vi "MAIN - TLB` Springboard Tool.vi"() -> ()   [LabVIEW 2014, in "TLB` Springboard.lvlib"]
uses:
  TLB` Springboard.lvlib
  Components/State Declaration.ctl
  Components/System Triggers.ctl
  <vilib>/Utility/error.llb/DialogTypeEnum.ctl
  <vilib>/NI/AMC/Read Termination Message.vi
  <vilib>/NI/AMC/Create Single Message.vi
  <vilib>/NI/AMC/Update Message Routing Info.vi
  <vilib>/NI/AMC/Create Multiple Messages.vi
  Components/TypeDef - SHIFTER - TLB` Springboard.ctl
  <vilib>/NI/AMC/Globals.vi
  <vilib>/NI/AMC/Send Message.vi
  Components/Dependencies.llb/TLB`_Dependencies.lvlib
  <vilib>/NI/AMC/AMC.lvlib
panel:
  in  "Add to Project":u16(ring) items=["< Create In New Project... >"]
  in  "Cancel":bool
  in  "Build":bool
  in  "New TLB Name":string
  in  "Destination Folder":path
  out "error out":errorcluster
  # "TLB` Springboard"
  # "Description"
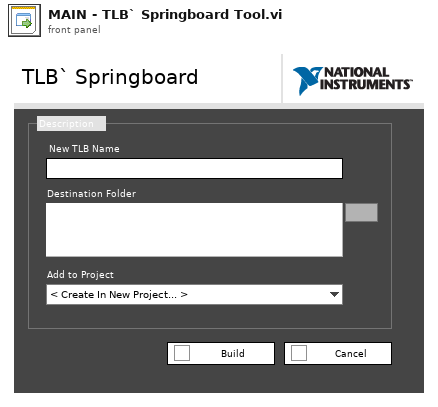
[diagram p1: front panel]
types:
  T1 = typedef "TLB` Springboard.lvlib/System Triggers.ctl" = enum16{"<None>", "Create New", "Cache User Parameters", "Close Application"}
  T2 = typedef "TLB` Springboard.lvlib/State Declaration.ctl" = enum16{"<Startup>", "Idle", "Creating", "<Shutdown>"}
  T3 = enum16{"Clear SR", "Set Display", "Set Shifter", "Initialize Events", "Init Q"}
  T4 = typedef "TLB` Springboard.lvlib/TypeDef - SHIFTER - TLB` Springboard.ctl" = cluster{"State":T2, "User Data":cluster{"New TLB Name":string, "Destination Folder":path, "Project Selection":u16}, "Display Data":cluster{"Active Item Tag":string}, "User Parameter Controls":refnum<vi>[], "Framework Data":cluster{"Exit Event":T5, "Terminate Error":errorcluster}, "Private Data":cluster{"Projects In Memory":refnum<vi>[], "Build Complete":bool}}
  T5 = typedef "TLB` Springboard.lvlib/TLB`_Dependencies.lvlib/Exit Event Ref.ctl" = refnum<user-event>
  T6 = typedef "AMC.lvlib/Message Queue.ctl" = refnum<queue>
  T7 = typedef "DialogTypeEnum.ctl" = enum16{"no dialog", "OK message", "continue or stop message", "auto error handling dialog", "OK message + warnings", "continue/stop + warnings"}
  T8 = enum8{"Enabled", "Disabled", "Disabled and Grayed Out"}
  T9 = enum32{"Invalid", "Standard", "Closed", "Hidden", "Minimized", "Maximized"}
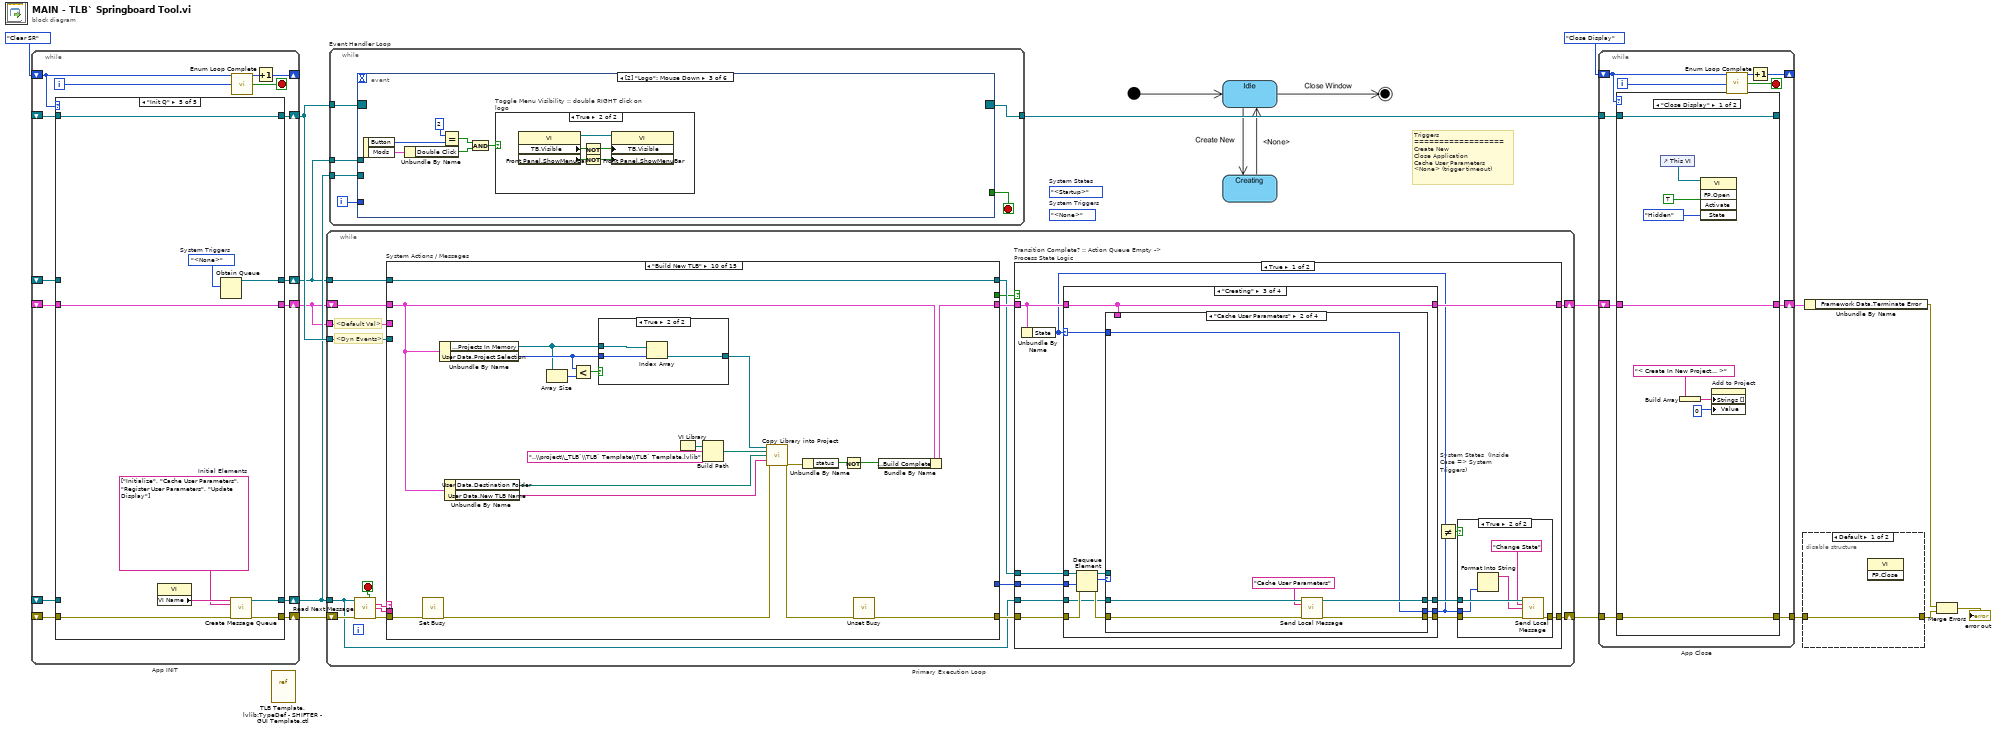
[diagram p0: block diagram]
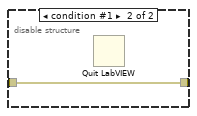
[diagram p2: hidden frame]
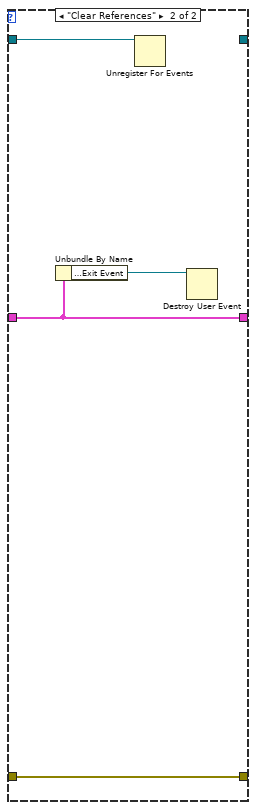
[diagram p3: hidden frame]
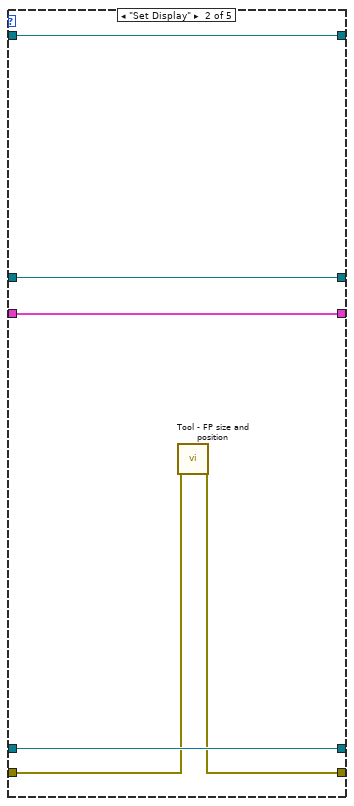
[diagram p5: hidden frame]
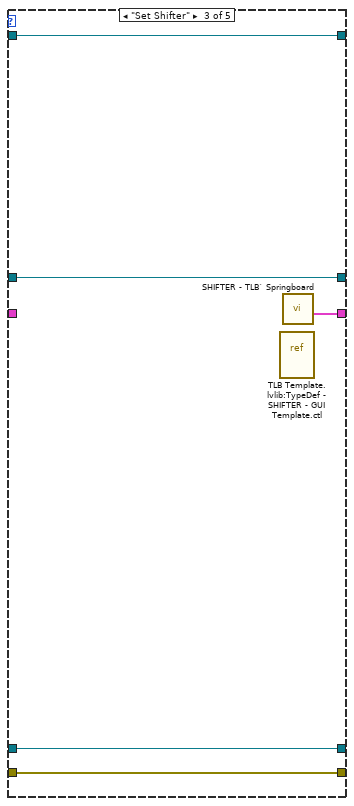
[diagram p6: hidden frame]
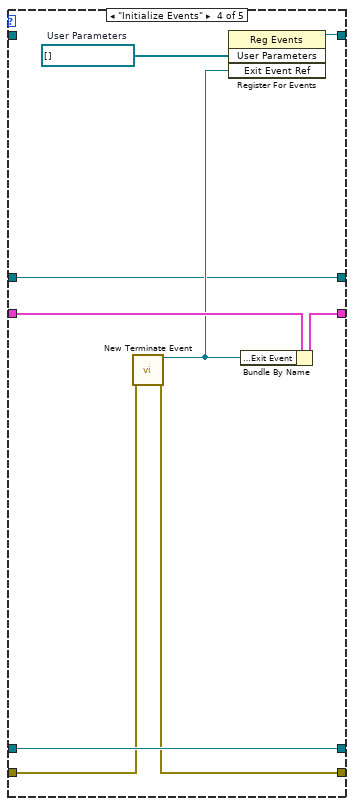
[diagram p7: hidden frame]
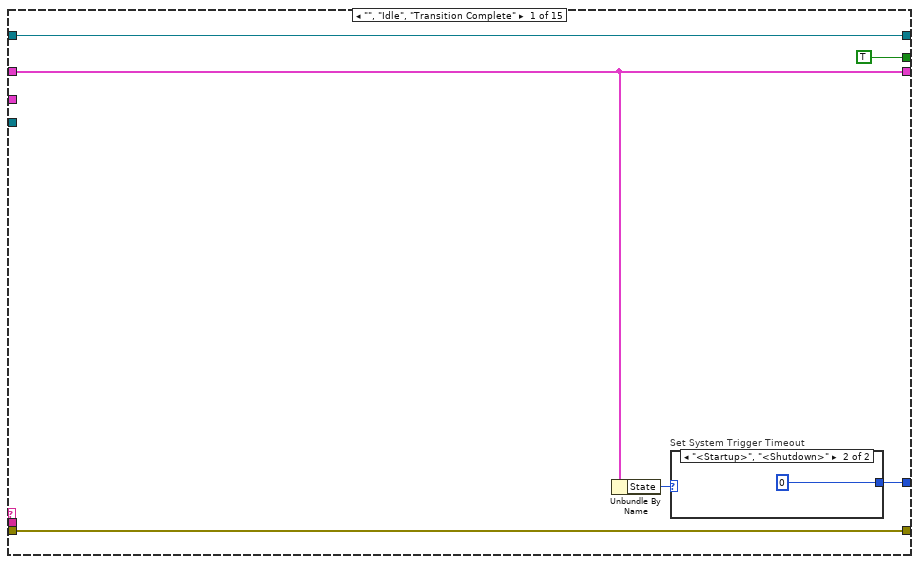
[diagram p8: hidden frame]
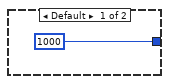
[diagram p9: hidden frame]
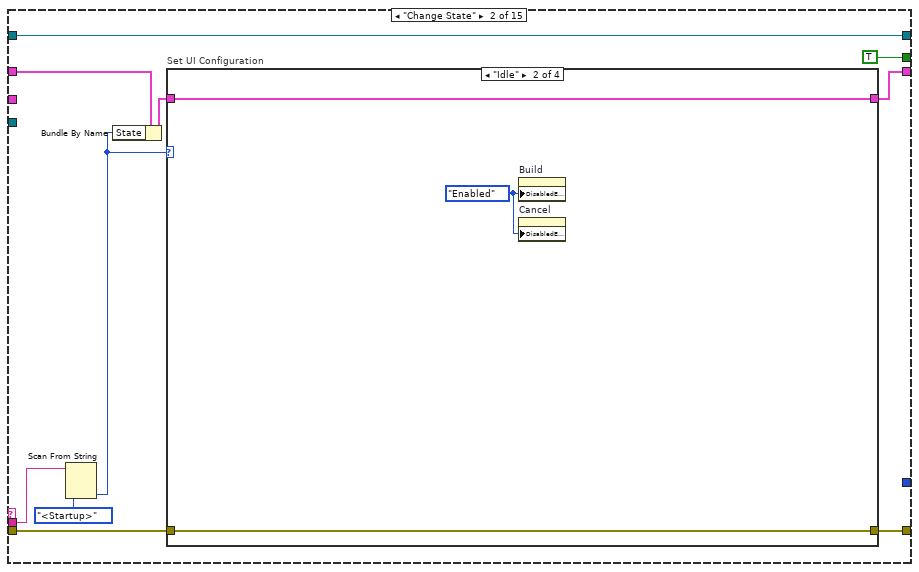
[diagram p10: hidden frame]
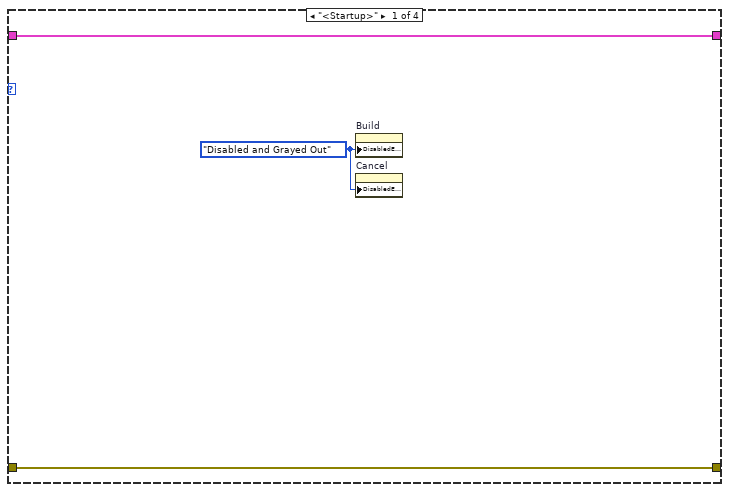
[diagram p11: hidden frame]
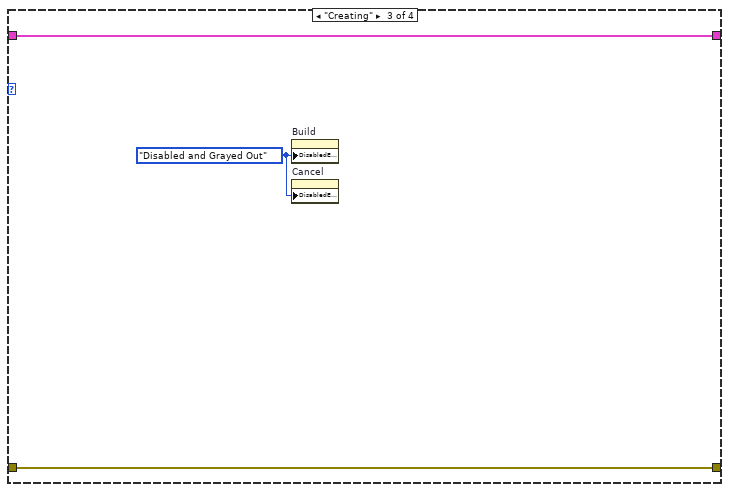
[diagram p12: hidden frame]
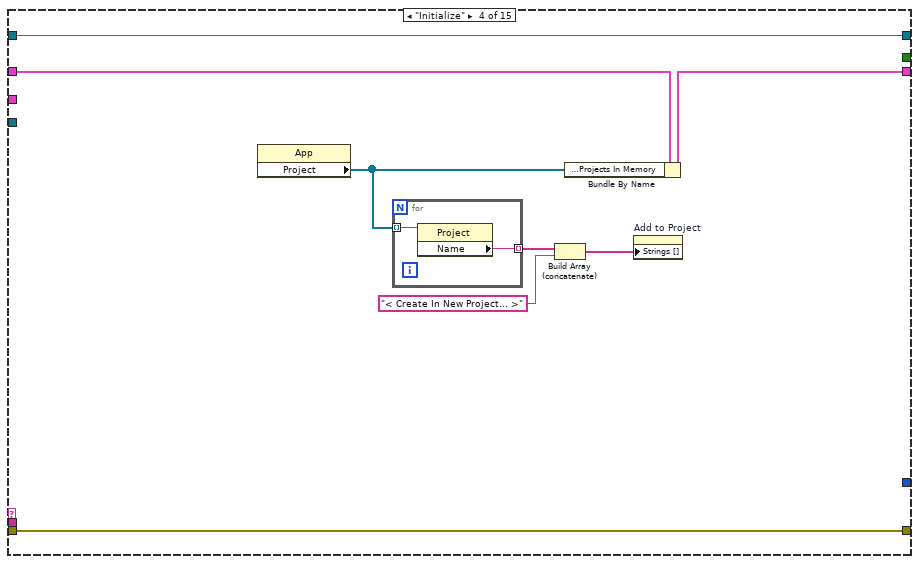
[diagram p15: hidden frame]
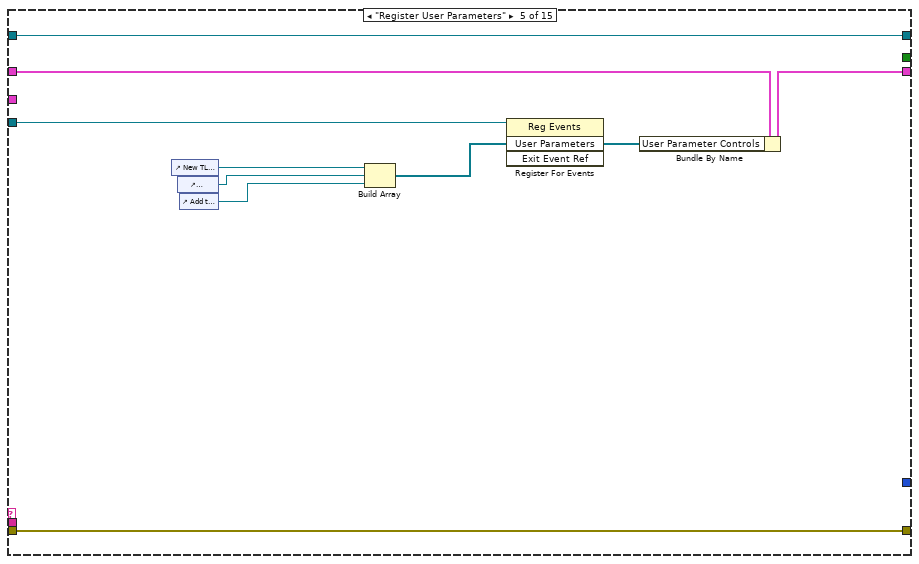
[diagram p16: hidden frame]
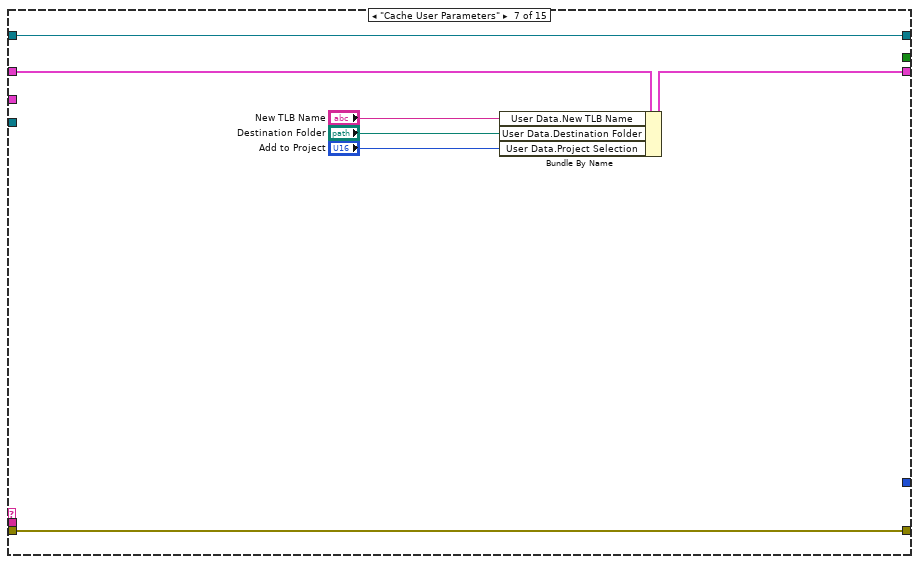
[diagram p18: hidden frame]
diagram:
  (unwired) System_Triggers."<None>"  # System Triggers
  (unwired) State_Declaration."<Startup>"  # System States
  # "Triggers\n==================\nCreate New\nClose Application\nCache User Parameters\n<None> (trigger timeout)"
  n1 = while "App INIT" {
    shift-right: [w23] -> _
    shift-left: T3."Clear SR" -> [w18]
    shift-right: [w29] -> w9
    shift-left: _ -> [w22]
    shift-right: [w26] -> w8
    shift-left: _ -> [w21]
    shift-right: [w28] -> w11
    shift-left: _ -> [w20]
    shift-right: [w27] -> w1
    shift-left: _ -> [w19]
    shift-right: [w17] -> w2
    shift-left: _ -> [w16]
    i -> [w24]
    stop <- w25 stop-if-true
    n2 = case shown="\"Init Q\"" w18 {
      tunnel: [_ w33 w40 w49 w55] -> w29
      tunnel: [_ w31 w39 w42 w53] -> w26
      tunnel: [_ w35 w36 w46 w57] -> w27
      tunnel: [_ w34 w38 w45 w58] -> w28
      tunnel: w22 -> [_ w33 w40 w49 _]
      tunnel: w21 -> [_ w32 w39 w43 w54]
      tunnel: w20 -> [_ w34 w38 _ w58]
      tunnel: w19 -> [_ w35 _ w47 w57]
      tunnel: [_ w30 w37 w41 w51] -> w17
      tunnel: w16 -> [_ w30 w37 w41 _]
      frame "Clear SR" {
      }
      frame "Set Display" {
        n3 = call "Tool - FP size and position.vi"("error in (no error)"=w32) -> ("error out"=w31:errorcluster)  [unwired: 7 in, 11 out]
      }
      frame "Set Shifter" {
        n4 = vi-ref "TLB Template.lvlib:TypeDef - SHIFTER - GUI Template.ctl"() -> ()  [unwired: 1 out]
        n5 = call "SHIFTER - TLB` Springboard.vi"() -> ("SHIFTER DATA"=w36:T4)  [unwired: 15 in]
      }
      frame "Initialize Events" {
        w48 = refnum<vi>[] []  # User Parameters
        n6 = call "New Terminate Event.vi"("error in (no error)"=w43) -> ("Exit Event Ref"=w44:T5, "error out"=w42:errorcluster)  [unwired: 13 in]
        n7 = register-events(w48, w44) -> (reference out=w45:refnum<event-registration>)  [unwired: 2 in, 1 out]
        n8 = Bundle By Name(cluster=w47, "Framework Data.Exit Event"=w44) -> (w46:T4)
      }
      frame "Init Q" {
        w50 = System_Triggers."<None>"  # System Triggers
        w52 = string[] ["Initialize", "Cache User Parameters", "Register User Parameters", "Update Display"]  # Initial Elements
        n9 = property class="VI"() -> ("VI Name"=w56:string)  [unwired: 2 in, 2 out]
        n10 = Obtain Queue(element data type=w50) -> (queue out=w51:refnum<queue>)  [unwired: 4 in, 2 out]
        n11 = call <vilib>:"Create Message Queue.vi"("message queue name"=w56, "initial message names"=w52, "error in"=w54) -> ("message queue out"=w55:T6, "error out"=w53:errorcluster)  [unwired: 11 in]
      }
    }
    n12 = call "Enum Loop Complete.vi"("Current State Enum"=w18, "Itteration"=w24) -> ("Loop Complete?"=w25:bool)  [unwired: 13 out]
    n13 = Increment(x=w18) -> (x+1=w23:T3)
  }
  n14 = vi-ref "TLB Template.lvlib:TypeDef - SHIFTER - GUI Template.ctl"() -> ()  [unwired: 1 out]
  n15 = while "Primary Execution Loop" {
    shift-right: [w65] -> w15
    shift-left: w8 -> [w72]
    shift-right: [w68] -> w14
    shift-left: w1 -> [w75]
    tunnel: w1 -> [w74]
    tunnel: w9 -> [w63]
    tunnel: w11 -> [w73]
    tunnel: w2 -> [w64]
    stop <- w70 stop-if-true
    # "<Dyn Events>"
    # "<Default Val>"
    n16 = call <vilib>:"Read Next Message.vi"("message queue in"=w63, "error in"=w72) -> ("exit process?"=w70:bool, "message name"=w69:string, "message value"=w60:string, "error out"=w71:errorcluster)  [unwired: 6 in, 4 out]
    n17 = case "System Actions / Messages" shown="\"Build New TLB\"" w69 {
      selector: w69 -> [_ _ _ _ _ _ _ _ _ _ _ _ _ _ w206]
      tunnel: [w81 w88 w107 w113 w126 w129 w134 w139 w142 w146 w169 w174 w196 w200 w210] -> w66
      tunnel: w71 -> [w81 w87 w107 w113 w126 w129 w134 w139 w142 w156 w169 w175 w196 w199 w211]
      tunnel: w75 -> [w76 w84 w106 w115 w125 w128 w136 w138 w141 w145 w168 w172 w195 w203 w212]
      tunnel: w74 -> [_ _ _ _ _ _ _ _ _ _ _ _ _ _ _]
      tunnel: [w76 w86 w106 w110 w124 w128 w135 w138 w141 w144 w168 w173 w195 w203 w212] -> w67
      tunnel: [w77 _ _ _ _ _ _ _ _ _ _ _ _ _ _] -> w59
      tunnel: w73 -> [_ _ _ _ w123 _ _ _ _ _ _ _ _ _ _]
      tunnel: [w79 w92 w105 w114 w122 w127 w133 w137 w140 w161 w167 w170 w194 w197 w204] -> w62
      tunnel: w64 -> [w79 w92 w105 w114 w122 w127 w133 w137 w140 w161 w167 w170 w194 w197 w204]
      tunnel: [TRUE TRUE _ _ _ _ _ _ _ _ _ _ _ _ _] -> w61
      tunnel: w60 -> [_ w91 _ _ _ _ _ _ _ _ _ _ _ _ _]
      frame "", "Idle", "Transition Complete" {
        n18 = Unbundle By Name(w76) -> ("State"=w78:T2)
        n19 = case "Set System Trigger Timeout" shown="\"<Startup>\", \"<Shutdown>\"" w78 {
          tunnel: [1000 0] -> w77
          frame Default {
          }
          frame "<Startup>", "<Shutdown>" {
          }
        }
      }
      frame "Change State" {
        n20 = Scan From String(input string=w91, default 1=State_Declaration."<Startup>" ("State")) -> (output 1=w89:T2)  [unwired: 3 in, 3 out]
        n21 = Bundle By Name(cluster=w84, "State"=w89) -> (w85:T4)
        n22 = case "Set UI Configuration" shown="\"Idle\"" w89 {
          tunnel: [w95 w99 w102 w104] -> w88
          tunnel: w87 -> [w95 w99 w102 w104]
          tunnel: [w96 w98 w101 w103] -> w86
          tunnel: w85 -> [w96 w98 w101 w103]
          frame "<Startup>" {
            w94 = T8."Disabled and Grayed Out" ("Disabled")
            n23 = property on="Build" class="Bool"("DisabledEnum"=w94) -> ()  [unwired: 2 in, 2 out]
            n24 = property on="Cancel" class="Bool"("DisabledEnum"=w94) -> ()  [unwired: 2 in, 2 out]
          }
          frame "Idle" {
            w97 = T8."Enabled" ("Disabled")
            n25 = property on="Build" class="Bool"("DisabledEnum"=w97) -> ()  [unwired: 2 in, 2 out]
            n26 = property on="Cancel" class="Bool"("DisabledEnum"=w97) -> ()  [unwired: 2 in, 2 out]
          }
          frame "Creating" {
            w100 = T8."Disabled and Grayed Out" ("Disabled")
            n27 = property on="Build" class="Bool"("DisabledEnum"=w100) -> ()  [unwired: 2 in, 2 out]
            n28 = property on="Cancel" class="Bool"("DisabledEnum"=w100) -> ()  [unwired: 2 in, 2 out]
          }
          frame "<Shutdown>" {
          }
        }
      }
      frame "/*********Initialize********/" {
      }
      frame "Initialize" {
        n29 = property class="App"() -> ("Project"=w109:refnum<vi>[])  [unwired: 2 in, 2 out]
        n30 = for {
          tunnel: w109 -> [w117] mode=indexing
          tunnel: [w116] -> w112 mode=indexing
          n31 = property class="Project"(reference=w117) -> ("Name"=w116:string)  [unwired: 1 in, 2 out]
        }
        n32 = Build Array (concatenate)(w112, "< Create In New Project... >") -> (w108:string[])
        n33 = Bundle By Name(cluster=w115, "Private Data.Projects In Memory"=w109) -> (w110:T4)
        n34 = property on="Add to Project" class="Ring (strict)"("Strings []"=w108) -> ()  [unwired: 2 in, 2 out]
      }
      frame "Register User Parameters" {
        n35 = control-ref of="New TLB Name"() -> (w120:refnum<vi>)
        n36 = control-ref of="Destination Folder"() -> (w118:refnum<vi>)
        n37 = control-ref of="Add to Project"() -> (w119:refnum<vi>)
        n38 = Build Array(w120, w118, w119) -> (w121:refnum<vi>[])
        n39 = register-events(reference=w123, w121) -> ()  [unwired: 2 in, 2 out]
        n40 = Bundle By Name(cluster=w125, "User Parameter Controls"=w121) -> (w124:T4)
      }
      frame "/*********Display Updates********/" {
      }
      frame "Cache User Parameters" {
        n41 = Bundle By Name(cluster=w136, "User Data.New TLB Name"="New TLB Name", "User Data.Destination Folder"="Destination Folder", "User Data.Project Selection"="Add to Project") -> (w135:T4)
      }
      frame "Update Display" {
      }
      frame "/*********Primary Execution********/" {
      }
      frame "Build New TLB" {
        n42 = call <vilib>:"Set Busy.vi"("error in (no error)"=w156) -> ("error out"=w151:errorcluster)  [unwired: 9 in, 1 out]
        n43 = Unbundle By Name(w145) -> ("Private Data.Projects In Memory"=w158:refnum<vi>[], "User Data.Project Selection"=w160:u16)
        n44 = Unbundle By Name(w145) -> ("User Data.Destination Folder"=w153:path, "User Data.New TLB Name"=w152:string)
        n45 = Array Size(array=w158) -> (size(s)=w159:i32)
        n46 = Less?(x=w160, y=w159) -> (x < y?=w157:bool)
        n47 = case shown="True" w157 {
          tunnel: w160 -> [_ w166]
          tunnel: w158 -> [_ w165]
          tunnel: [w162 w164] -> w155
          frame False {
            n48 = invoke class="App" method="Project.New"() -> ("Project:New"=w163:refnum<vi>)  [unwired: 3 in, 2 out]
            n49 = invoke class="Project" method="Open Window"(reference=w163) -> (reference out=w162:refnum<vi>)  [unwired: 2 in, 2 out]
          }
          frame True {
            n50 = Index Array(array=w165, index=w166) -> (element=w164:refnum<vi>)
          }
        }
        n51 = VI Library() -> (path=w150:path)
        n52 = Build Path(base path=w150, name or relative path="..\\project\\_TLB`\\TLB` Template\\TLB` Template.lvlib") -> (appended path=w154:path)
        n53 = call "Copy Library into Project.vi"("Project"=w155, "Library Path"=w154, "Destination Folder"=w153, "New TLB Name"=w152, "error in"=w151) -> ("error out"=w148:errorcluster)  [unwired: 10 in]
        n54 = Unbundle By Name(w148) -> ("status"=w147:bool)
        n55 = Not(x=w147) -> (.not. x?=w143:bool)
        n56 = call <vilib>:"Unset Busy.vi"("error in (no error)"=w148) -> ("error out"=w146:errorcluster)  [unwired: 10 in]
        n57 = Bundle By Name(cluster=w145, "Private Data.Build Complete"=w143) -> (w144:T4)
      }
      frame "/*********Shutdown********/" {
      }
      frame "Error" {
        n58 = Unbundle By Name(w172) -> ("State"=w171:T2)
        n59 = case shown="Default" w171 {
          tunnel: w175 -> [w183]
          tunnel: [w182] -> w174
          tunnel: w172 -> [w179]
          tunnel: [w178] -> w173
          tunnel: w170 -> [w176]
          frame Default {
            n60 = call <vilib>:"General Error Handler CORE.vi"("type of dialog (OK msg:1)"=DialogTypeEnum."auto error handling dialog", "error in (no error)"=w183) -> ("stop event propagated"=w181:bool, "error out"=w177:errorcluster)  [unwired: 12 out]
            n61 = case "User Chose to Stop and Not Continue\nFALSE = Continue: CLEAR ERRORS" shown="True" w181 {
              tunnel: [w184 w188] -> w182
              tunnel: w177 -> [w185 w191]
              tunnel: w179 -> [w186 w193]
              tunnel: [w186 w192] -> w178
              tunnel: w176 -> [_ w189]
              frame False {
                n62 = call <vilib>:"Clear Errors.vi"("error in (no error)"=w185) -> ("error out"=w184:errorcluster)  [unwired: 1 in, 5 out]
              }
              frame True {
                n63 = call <vilib>:"Clear Errors.vi"("error in (no error)"=w191) -> ("error out"=w187:errorcluster)  [unwired: 1 in, 5 out]
                n64 = Bundle By Name(cluster=w193, "Framework Data.Terminate Error"=w191) -> (w192:T4)
                n65 = Enqueue Element(queue=w189, element=System_Triggers."Close Application", error in (no error)=w187) -> (error out=w188:errorcluster)  [unwired: 1 in, 2 out]
              }
            }
          }
        }
      }
      frame "Close Window" {
      }
      frame "Exit" {
        w198 = refnum<class> refnum  # event data
        # "Don't wire 'Error In'\nMust Execute Regardless"
        n66 = Unbundle By Name(w203) -> ("Framework Data.Exit Event"=w202:T5)
        n67 = Generate User Event(user event=w202, event data cluster=w198) -> (error out=w201:errorcluster)  [unwired: 2 in, 1 out]
        n68 = Merge Errors(w201, w199) -> (w200:errorcluster)
      }
      frame Default {
        w208 = 1 items=["No error", "Argument error", "Memory is full", "Out of zone", "End of file", "File already open", "Generic file I/O error", "File not found", "File permission error", "Disk is full", "Duplicate path", "Too many files open", "System feature not enabled", "Resource file not found", "Cannot add resource", "Resource not found", "Image not found", "Image memory error", "Pen does not exist", "Config type invalid", "Config token not found", "Config parse error", "Config memory error", "Bad external code format", "Bad external code offset", "External code not present", "Null window", "Destroy window error", "Null menu", "Print aborted", "Bad print record", "Print driver error", "Windows error during printing", "Memory error during printing", "Print dialog error", "Generic print error", "Invalid device refnum", "Device not found", "Device parameter error", "Device unit error", "Cannot open device", "Device call aborted", "Generic error", "Cancelled by user", "Object ID too low", "Object ID too high", "Object not in heap", "Unknown heap", "Unknown object (invalid DefProc)", "Unknown object (DefProc not in table)", "Message out of range", "Invalid (null) method", "Unknown message", "Manager call not supported", "Bad address", "Network operation in progress", "Network operation timed out", "Connection is busy", "Network attribute not supported", "Network error", "Address in use", "System out of memory", "Connection aborted", "Connection refused", "Not connected", "Already connected", "Connection closed", "Initialization error (interapplication manager)", "Bad occurrence", "Wait on unbound occurrence handler", "Occurrence queue overflow", "Datalog type conflict", "Unused", "Unrecognized type (interapplication manager)", "Memory corrupt", "Failed to make temporary DLL", "Old CIN version", "Drag socket not found", "Failed to load drop-object", "Failed to register OLE object", "Failed to release OLE object", "Format specifier type mismatch", "Unknown format specifier", "Too few format specifiers", "Too many format specifiers", "Scan failed", "Newer CIN version", "Error converting to variant", "Runtime menu error", "Password tampered", "Variant attribute not found", "Incompatible variant data type", "Event data is not available", "Event Store is not present", "Occurrence is not found", "Event Queue is not created", "Event info is not available", "Refnum passed is NULL", "Error retrieving Class GUID", "Error retrieving CoClass GUID", "Error retrieving TypeLib GUID.", "Bad built application magic bytes.", "Specific driver is different from the specific driver associated with the Logical Name.", "There is no session opened to the class driver.", "Max Error", "MAX - Error with config objects", "MAX - Error loading configuration", "MAX - Group not supported"]
        w209 = TRUE  # status
        n69 = Format Into String(format string="DEVELOPER ERROR:\nImproper State Requested\n================\nState {%s} does not exist within this architecture\n\nCheck for spelling and case errors" ("source"), w206) -> (resulting string=w207:string)  [unwired: 2 in, 1 out]
        n70 = Bundle By Name(cluster=w211, "status"=w209, "code"=w208, "source"=w207) -> (w210:errorcluster)
      }
    }
    n71 = case "Transition Complete? :: Action Queue Empty -> Process State Logic" shown="True" w61 {
      tunnel: [w224 w330] -> w68
      tunnel: w67 -> [w214 w330]
      tunnel: w66 -> [w223 w329]
      tunnel: w63 -> [w222 _]
      tunnel: [w218 w329] -> w65
      tunnel: w62 -> [w221 _]
      tunnel: w59 -> [w215 _]
      frame True {
        n72 = Unbundle By Name(w214) -> ("State"=w213:T2)
        n73 = case "System States  (Inside Case => System Triggers)" shown="\"Creating\"" w213 {
          selector: w213 -> [_ w249 w279 _]
          tunnel: [w240 w248 w289 w320] -> w224
          tunnel: w214 -> [w240 w248 w289 w320]
          tunnel: w223 -> [w234 w253 w283 w314]
          tunnel: w222 -> [w232 w251 w281 w312]
          tunnel: [w239 w258 w288 w319] -> w219
          tunnel: w221 -> [w242 w246 w290 w322]
          tunnel: [w238 w257 w287 w318] -> w220
          tunnel: [w237 w256 w286 w317] -> w217
          tunnel: w215 -> [w236 w254 w284 w316]
          frame "<Startup>" {
            n74 = Dequeue Element(queue=w242, timeout in ms (-1)=w236, error in (no error)=w234) -> (queue out=w235:refnum<queue>, element=w241:T1, error out=w233:errorcluster)  [unwired: 1 out]
            n75 = case shown="\"<None>\", Default" w241 {
              tunnel: w240 -> [_]
              tunnel: [w244] -> w239
              tunnel: w233 -> [w244]
              tunnel: w232 -> [w245]
              tunnel: [w245] -> w238
              tunnel: [State_Declaration."Idle" ("State")] -> w237
              tunnel: w235 -> [_]
              frame "<None>", Default {
              }
            }
          }
          frame "Idle" {
            n76 = Dequeue Element(queue=w246, timeout in ms (-1)=w254, error in (no error)=w253) -> (queue out=w250:refnum<queue>, element=w255:T1, error out=w252:errorcluster)  [unwired: 1 out]
            n77 = case shown="\"Cache User Parameters\"" w255 {
              tunnel: w248 -> [_ _ _ _ _]
              tunnel: [w261 w265 w268 w271 w275] -> w258
              tunnel: w252 -> [w261 w265 w268 w271 w278]
              tunnel: w251 -> [w262 w264 w269 w272 w277]
              tunnel: [w262 w264 w269 w272 w276] -> w257
              tunnel: [State_Declaration."Idle" ("State") State_Declaration."Creating" ("State") State_Declaration."<Shutdown>" ("State") State_Declaration."Idle" ("State") w273] -> w256
              tunnel: w250 -> [_ _ _ _ _]
              tunnel: w249 -> [_ _ _ _ w273]
              frame "<None>" {
              }
              frame "Create New" {
              }
              frame "Close Application" {
              }
              frame Default {
              }
              frame "Cache User Parameters" {
                n78 = call <vilib>:"Send Local Message.vi"("message queue in"=w277, "message name"="Cache User Parameters" ("Message Name"), "error in"=w278) -> ("message queue out"=w276:T6, "error out"=w275:errorcluster)  [unwired: 10 in, 1 out]
              }
            }
            n79 = Unbundle By Name(w248) -> ("Private Data.Build Complete"=w247:bool)
            n80 = case shown="True" w247 {
              tunnel: w246 -> [_ w259]
              frame False {
              }
              frame True {
                n81 = Enqueue Element(queue=w259, element=System_Triggers."Close Application" ("System Triggers")) -> ()  [unwired: 2 in, 3 out]
              }
            }
          }
          frame "Creating" {
            n82 = Dequeue Element(queue=w290, timeout in ms (-1)=w284, error in (no error)=w283) -> (queue out=w280:refnum<queue>, element=w285:T1, error out=w282:errorcluster)  [unwired: 1 out]
            n83 = case shown="\"Cache User Parameters\"" w285 {
              tunnel: w289 -> [_ _ _ _]
              tunnel: [w294 w299 w303 w307] -> w288
              tunnel: w282 -> [w295 w302 w303 w308]
              tunnel: w281 -> [w293 w301 w304 w306]
              tunnel: [w292 w300 w304 w306] -> w287
              tunnel: [State_Declaration."Idle" ("State") w297 State_Declaration."Creating" ("State") State_Declaration."Idle" ("State")] -> w286
              tunnel: w280 -> [_ _ _ w310]
              tunnel: w279 -> [_ w297 _ _]
              frame "<None>" {
                n84 = call <vilib>:"Send Local Message.vi"("message queue in"=w293, "message name"="Build New TLB" ("Message Name"), "error in"=w295) -> ("message queue out"=w292:T6, "error out"=w294:errorcluster)  [unwired: 10 in, 1 out]
              }
              frame "Cache User Parameters" {
                n85 = call <vilib>:"Send Local Message.vi"("message queue in"=w301, "message name"="Cache User Parameters" ("Message Name"), "error in"=w302) -> ("message queue out"=w300:T6, "error out"=w299:errorcluster)  [unwired: 10 in, 1 out]
              }
              frame Default {
              }
              frame "Close Application" {
                n86 = Enqueue Element(queue=w310, element=System_Triggers."Close Application" ("System Triggers"), error in (no error)=w308) -> (error out=w307:errorcluster)  [unwired: 1 in, 2 out]
              }
            }
          }
          frame "<Shutdown>" {
            n87 = Dequeue Element(queue=w322, timeout in ms (-1)=w316, error in (no error)=w314) -> (queue out=w315:refnum<queue>, element=w321:T1, error out=w313:errorcluster)  [unwired: 1 out]
            n88 = case shown="\"<None>\", Default" w321 {
              tunnel: w320 -> [_]
              tunnel: [w323] -> w319
              tunnel: w313 -> [w325]
              tunnel: w312 -> [w326]
              tunnel: [w324] -> w318
              tunnel: [State_Declaration."<Shutdown>" ("State")] -> w317
              tunnel: w315 -> [_]
              frame "<None>", Default {
                n89 = call <vilib>:"Send Local Messages.vi"("message queue in"=w326, "message names"=string[] ["Exit"], "error in"=w325) -> ("message queue out"=w324:T6, "error out"=w323:errorcluster)  [unwired: 10 in, 1 out]
              }
            }
          }
        }
        n90 = Not Equal?(x=w213, y=w217) -> (x != y?=w216:bool)
        n91 = case shown="True" w216 {
          tunnel: w220 -> [_ w231]
          tunnel: w219 -> [w225 w230]
          tunnel: [w225 w229] -> w218
          tunnel: w217 -> [_ w227]
          frame False {
          }
          frame True {
            n92 = Format Into String(w227) -> (resulting string=w226:string)  [unwired: 3 in, 1 out]
            n93 = call <vilib>:"Send Local Message.vi"("message queue in"=w231, "message name"="Change State" ("Message Name"), "message value"=w226, "error in"=w230) -> ("error out"=w229:errorcluster)  [unwired: 9 in, 2 out]
          }
        }
      }
      frame False {
      }
    }
  }
  n94 = while "Event Handler Loop" {
    tunnel: w11 -> [w335]
    tunnel: w9 -> [w334]
    tunnel: [w333] -> w13
    tunnel: w2 -> [w331]
    i -> [w332]
    stop <- w336 stop-if-true
    n95 = event shown="[2] \"Logo\": Mouse Down" {
      selector: w335 -> [_ _ _ _ _ _]
      dyn-events: [_ _ _ _ _ _] -> w333
      timeout: _ -> [_ _ _ _ _ _]
      tunnel: [_ _ _ TRUE ("NewVal") _ _] -> w336
      tunnel: w334 -> [_ _ _ _ _ _]
      tunnel: w332 -> [_ _ _ _ _ _]
      tunnel: w331 -> [w338 w341 _ w354 w358 w360]
      event Panel Close? {
        w339 = TRUE  # Discard?
        n96 = event-data() -> ()  [unwired: 2 out]
        n97 = Enqueue Element(queue=w338, element=System_Triggers."Close Application") -> ()  [unwired: 2 in, 3 out]
        n98 = event-data("Discard?"=w339) -> ()  [unwired: 1 in, 1 out]
      }
      event "Cancel": Value Change {
        n99 = event-data() -> ()  [unwired: 4 out]
        n100 = Enqueue Element(queue=w341, element=System_Triggers."Close Application") -> ()  [unwired: 2 in, 3 out]
      }
      event Mouse Down {
        n101 = event-data() -> ("Button"=w346:u16, "Mods"=w347:cluster{"Double Click":bool, "Menu Key":bool})  [unwired: 1 out]
        n102 = Unbundle By Name(w347) -> ("Double Click"=w343:bool)
        n103 = Equal?(x=u16 2, y=w346) -> (x = y?=w344:bool)
        n104 = And(x=w344, y=w343) -> (x .and. y?=w342:bool)
        n105 = case "Toggle Menu Visibility :: double RIGHT click on logo" shown="True" w342 {
          frame False {
          }
          frame True {
            n106 = property class="VI"() -> (reference out=w352:refnum<vi>, "TB.Visible"=w350:bool, "Front Panel.ShowMenuBar"=w349:bool)  [unwired: 2 in, 1 out]
            n107 = Not(x=w350) -> (.not. x?=w351:bool)
            n108 = Not(x=w349) -> (.not. x?=w348:bool)
            n109 = property class="VI"(reference=w352, "TB.Visible"=w351, "Front Panel.ShowMenuBar"=w348) -> ()  [unwired: 1 in, 2 out]
          }
        }
      }
      event User Event {
        w353 = System_Triggers."Close Application"  # System Triggers
        n110 = event-data() -> ()  [unwired: 2 out]
        n111 = Enqueue Element(queue=w354, element=w353) -> ()  [unwired: 2 in, 3 out]
      }
      event Value Change {
        n112 = event-data() -> ()  [unwired: 2 out]
        n113 = Enqueue Element(queue=w358, element=System_Triggers."Cache User Parameters") -> (queue out=w357:refnum<queue>)  [unwired: 2 in, 2 out]
        n114 = event "use this event case to register a SPEICIFIC 'User Parameter' for a SPECIFIC action" shown="[0] Timeout" {
          selector: _ -> [_]
          dyn-events: _ -> [_]
          timeout: 0 -> [_]
          tunnel: w357 -> [_]
          event Timeout {
            n115 = event-data() -> ()  [unwired: 1 in, 1 out]
          }
        }
      }
      event "Build": Value Change {
        n116 = event-data() -> ()  [unwired: 4 out]
        n117 = Enqueue Element(queue=w360, element=System_Triggers."Create New") -> ()  [unwired: 2 in, 3 out]
      }
    }
  }
  n118 = while "App Close" {
    shift-right: [w368] -> _
    shift-left: enum16{"Close Display", "Clear References"}."Close Display" -> [w367]
    tunnel: w13 -> [w365]
    tunnel: w15 -> [w366]
    tunnel: [w363] -> w7
    shift-right: [w362] -> w5
    shift-left: w14 -> [w364]
    i -> [w369]
    stop <- w370 stop-if-true
    n119 = case shown="\"Close Display\"" w367 {
      tunnel: [w378 w383] -> w363
      tunnel: [w377 w382] -> w362
      tunnel: [w379 _] -> _
      tunnel: w366 -> [w378 w383]
      tunnel: w365 -> [w379 w380]
      tunnel: w364 -> [w377 w382]
      frame "Close Display" {
        n120 = control-ref of="This VI"() -> (w371:refnum<vi>)
        n121 = Build Array("< Create In New Project... >") -> (w376:string[])
        n122 = invoke class="VI" method="FP.Open"(reference=w371, "Activate"=TRUE ("Activate?"), "State"=T9."Hidden") -> ()  [unwired: 2 in, 5 out]
        n123 = property on="Add to Project" class="Ring (strict)"("Strings []"=w376, "Value"=u16 0) -> ()  [unwired: 2 in, 2 out]
      }
      frame "Clear References" {
        n124 = Unbundle By Name(w382) -> ("Framework Data.Exit Event"=w381:T5)
        n125 = Unregister For Events(event registration refnum=w380) -> ()  [unwired: 1 in, 1 out]
        n126 = Destroy User Event(user event=w381) -> ()  [unwired: 1 in, 1 out]
      }
    }
    n127 = call "Enum Loop Complete.vi"("Current State Enum"=w367, "Itteration"=w369) -> ("Loop Complete?"=w370:bool)  [unwired: 13 out]
    n128 = Increment(x=w367) -> (x+1=w368:enum16{"Close Display", "Clear References"})
  }
  n129 = disable-structure shown="Default" {
    disable-tunnel: [w384 w385] -> w4
    disable-tunnel: w7 -> [w384 w385]
    frame condition #0 (active) {
      n130 = invoke class="VI" method="FP.Close"() -> ()  [unwired: 3 in, 3 out]
    }
    frame condition #1 {
      n131 = Quit LabVIEW() -> ()  [unwired: 1 in]
    }
  }
  n132 = Unbundle By Name(w5) -> ("Framework Data.Terminate Error"=w3:errorcluster)
  n133 = Merge Errors(w3, w4) -> (→"error out":errorcluster)
